vi "get extended settings.vi"(8 "error in (no error)":errorcluster, 10 "extended_settings":cluster{"Param1":u32}, 11 "id":i32) -> (0 "error out":errorcluster, 2 "extended_settings out":cluster{"Param1":u32}, 3 "function return":i32)   [LabVIEW 2012, in "libximc.lvlib"]
doc: "result_t XIMC_API get_extended_settings (device_t id, extended_settings_t* extended_settings);"
uses:
  libximc.lvlib
  libximc.dll
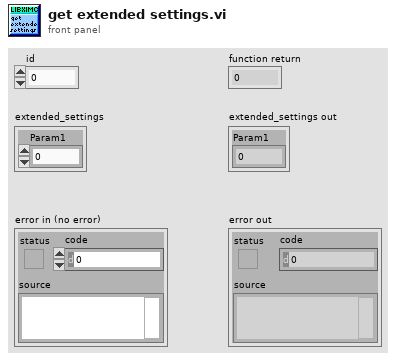
[diagram p1: front panel]
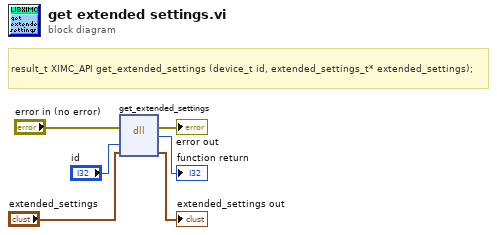
[diagram p0: block diagram]
diagram:
  # "result_t XIMC_API get_extended_settings (device_t id, extended_settings_t* extended_settings);"
  n1 = dll-call lib="E:/labview-2.12.1-Labview_12.0/ximcLVx32/libximc.*" fn="get_extended_settings"(error in="error in (no error)", "id"="id", "extended_settings"="extended_settings") -> (error out=→"error out":errorcluster, →"function return":i32, "extended_settings"=→"extended_settings out":cluster{"Param1":u32})  [unwired: 3 in, 1 out]
